vi "ASM.StateExecution.vi"(8 "error in (no error)":errorcluster, 11 "ActorStateMachine in":refnum<class "ActorStateMachine.lvclass">) -> (0 "error out":errorcluster, 3 "ActorStateMachine out":refnum<class "ActorStateMachine.lvclass">)   [LabVIEW 2021, in "ActorStateMachine.lvlib" / "ActorStateMachine.lvclass"]
uses:
  ActorStateMachine.lvclass
  ActorStateMachine.lvclass/ActorStateMachine.ctl
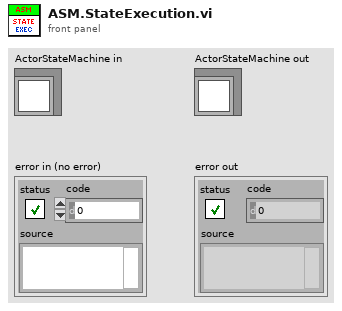
[diagram p1: front panel]
types:
  T1 = typedef "ActorStateMachine.lvlib/ActorStateMachine.lvclass/_ASM.State.ctl" = enum16{"Boom", "Pre-Init", "Init", "Post-Init", "Pre-Reset", "Reset", "Post-Reset", "Pre-Config", "Config", "Post-Config", "Pre-Ready", "Ready", "Post-Ready", "Pre-Running", "Running", "Next", "Post-Running", "Break", "Fail", "Crash", "Shutdown", "Doom"}
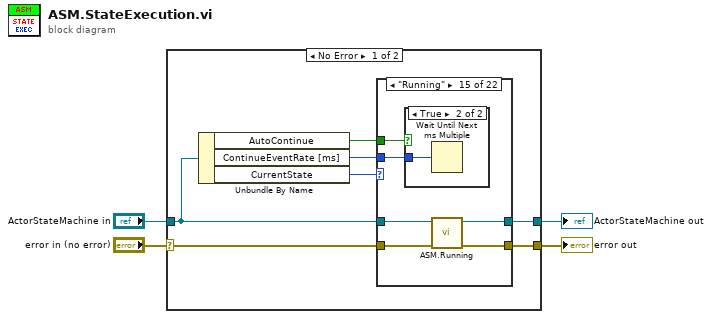
[diagram p0: block diagram]
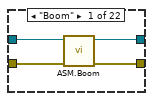
[diagram p2: hidden frame]
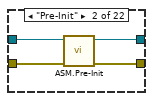
[diagram p3: hidden frame]
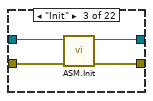
[diagram p4: hidden frame]
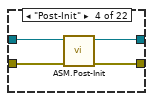
[diagram p5: hidden frame]
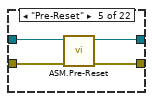
[diagram p6: hidden frame]
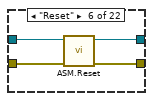
[diagram p7: hidden frame]
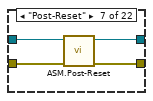
[diagram p8: hidden frame]
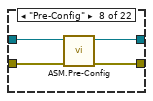
[diagram p9: hidden frame]
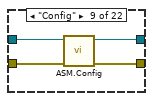
[diagram p10: hidden frame]
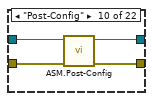
[diagram p11: hidden frame]
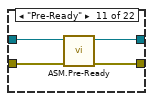
[diagram p12: hidden frame]
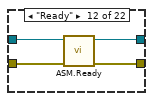
[diagram p13: hidden frame]
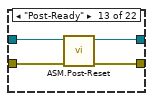
[diagram p14: hidden frame]
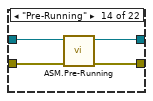
[diagram p15: hidden frame]
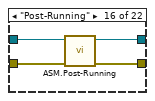
[diagram p17: hidden frame]
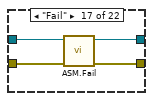
[diagram p18: hidden frame]
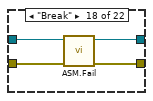
[diagram p19: hidden frame]
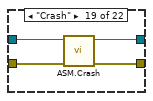
[diagram p20: hidden frame]
diagram:
  n1 = case shown="No Error" "error in (no error)" {
    selector: "error in (no error)" -> [w8 w102]
    tunnel: [w7 w102] -> w3
    tunnel: [w10 w101] -> w1
    tunnel: "ActorStateMachine in" -> [w9 w101]
    frame No Error {
      n2 = Unbundle By Name(w9) -> ("AutoContinue"=w5:bool, "ContinueEventRate [ms]"=w6:u32, "CurrentState"=w11:T1)
      n3 = case shown="\"Running\"" w11 {
        tunnel: [w14 w18 w23 w26 w30 w34 w38 w42 w46 w50 w54 w58 w62 w66 w70 w77 w81 w85 w89 w93 w97 w99] -> w7
        tunnel: [w12 w16 w21 w24 w28 w32 w36 w40 w44 w48 w52 w56 w60 w64 w71 w75 w79 w83 w87 w91 w95 w100] -> w10
        tunnel: w9 -> [w13 w17 w22 w25 w29 w33 w37 w41 w45 w49 w53 w57 w61 w65 w72 w76 w80 w84 w88 w92 w96 w100]
        tunnel: w8 -> [w15 w19 w20 w27 w31 w35 w39 w43 w47 w51 w55 w59 w63 w67 w73 w78 w82 w86 w90 w94 w98 w99]
        tunnel: w6 -> [_ _ _ _ _ _ _ _ _ _ _ _ _ _ w69 _ _ _ _ _ _ _]
        tunnel: w5 -> [_ _ _ _ _ _ _ _ _ _ _ _ _ _ w68 _ _ _ _ _ _ _]
        frame "Boom" {
          n4 = call-dynamic "ASM.Boom.vi"("error in (no error)"=w15, "ActorStateMachine in"=w13) -> ("error out"=w14:errorcluster, "ActorStateMachine out"=w12:refnum<class "ActorStateMachine.lvclass">)  [unwired: 8 in]
        }
        frame "Pre-Init" {
          n5 = call-dynamic "ASM.Pre-Init.vi"("error in (no error)"=w19, "ActorStateMachine in"=w17) -> ("error out"=w18:errorcluster, "ActorStateMachine out"=w16:refnum<class "ActorStateMachine.lvclass">)  [unwired: 8 in]
        }
        frame "Init" {
          n6 = call-dynamic "ASM.Init.vi"("error in (no error)"=w20, "ActorStateMachine in"=w22) -> ("error out"=w23:errorcluster, "ActorStateMachine out"=w21:refnum<class "ActorStateMachine.lvclass">)  [unwired: 8 in]
        }
        frame "Post-Init" {
          n7 = call-dynamic "ASM.Post-Init.vi"("error in (no error)"=w27, "ActorStateMachine in"=w25) -> ("error out"=w26:errorcluster, "ActorStateMachine out"=w24:refnum<class "ActorStateMachine.lvclass">)  [unwired: 8 in]
        }
        frame "Pre-Reset" {
          n8 = call-dynamic "ASM.Pre-Reset.vi"("error in (no error)"=w31, "ActorStateMachine in"=w29) -> ("error out"=w30:errorcluster, "ActorStateMachine out"=w28:refnum<class "ActorStateMachine.lvclass">)  [unwired: 8 in]
        }
        frame "Reset" {
          n9 = call-dynamic "ASM.Reset.vi"("error in (no error)"=w35, "ActorStateMachine in"=w33) -> ("error out"=w34:errorcluster, "ActorStateMachine out"=w32:refnum<class "ActorStateMachine.lvclass">)  [unwired: 8 in]
        }
        frame "Post-Reset" {
          n10 = call-dynamic "ASM.Post-Reset.vi"("error in (no error)"=w39, "ActorStateMachine in"=w37) -> ("error out"=w38:errorcluster, "ActorStateMachine out"=w36:refnum<class "ActorStateMachine.lvclass">)  [unwired: 8 in]
        }
        frame "Pre-Config" {
          n11 = call-dynamic "ASM.Pre-Config.vi"("error in (no error)"=w43, "ActorStateMachine in"=w41) -> ("error out"=w42:errorcluster, "ActorStateMachine out"=w40:refnum<class "ActorStateMachine.lvclass">)  [unwired: 8 in]
        }
        frame "Config" {
          n12 = call-dynamic "ASM.Config.vi"("error in (no error)"=w47, "ActorStateMachine in"=w45) -> ("error out"=w46:errorcluster, "ActorStateMachine out"=w44:refnum<class "ActorStateMachine.lvclass">)  [unwired: 8 in]
        }
        frame "Post-Config" {
          n13 = call-dynamic "ASM.Post-Config.vi"("error in (no error)"=w51, "ActorStateMachine in"=w49) -> ("error out"=w50:errorcluster, "ActorStateMachine out"=w48:refnum<class "ActorStateMachine.lvclass">)  [unwired: 8 in]
        }
        frame "Pre-Ready" {
          n14 = call-dynamic "ASM.Pre-Ready.vi"("error in (no error)"=w55, "ActorStateMachine in"=w53) -> ("error out"=w54:errorcluster, "ActorStateMachine out"=w52:refnum<class "ActorStateMachine.lvclass">)  [unwired: 8 in]
        }
        frame "Ready" {
          n15 = call-dynamic "ASM.Ready.vi"("error in (no error)"=w59, "ActorStateMachine in"=w57) -> ("error out"=w58:errorcluster, "ActorStateMachine out"=w56:refnum<class "ActorStateMachine.lvclass">)  [unwired: 8 in]
        }
        frame "Post-Ready" {
          n16 = call-dynamic "ASM.Post-Reset.vi"("error in (no error)"=w63, "ActorStateMachine in"=w61) -> ("error out"=w62:errorcluster, "ActorStateMachine out"=w60:refnum<class "ActorStateMachine.lvclass">)  [unwired: 8 in]
        }
        frame "Pre-Running" {
          n17 = call-dynamic "ASM.Pre-Running.vi"("error in (no error)"=w67, "ActorStateMachine in"=w65) -> ("error out"=w66:errorcluster, "ActorStateMachine out"=w64:refnum<class "ActorStateMachine.lvclass">)  [unwired: 8 in]
        }
        frame "Running" {
          n18 = case shown="True" w68 {
            tunnel: w69 -> [_ w74]
            frame False {
            }
            frame True {
              n19 = Wait Until Next ms Multiple(millisecond multiple=w74) -> ()  [unwired: 1 out]
            }
          }
          n20 = call-dynamic "ASM.Running.vi"("error in (no error)"=w73, "ActorStateMachine in"=w72) -> ("error out"=w70:errorcluster, "ActorStateMachine out"=w71:refnum<class "ActorStateMachine.lvclass">)  [unwired: 8 in]
        }
        frame "Post-Running" {
          n21 = call-dynamic "ASM.Post-Running.vi"("error in (no error)"=w78, "ActorStateMachine in"=w76) -> ("error out"=w77:errorcluster, "ActorStateMachine out"=w75:refnum<class "ActorStateMachine.lvclass">)  [unwired: 8 in]
        }
        frame "Fail" {
          n22 = call-dynamic "ASM.Fail.vi"("error in (no error)"=w82, "ActorStateMachine in"=w80) -> ("error out"=w81:errorcluster, "ActorStateMachine out"=w79:refnum<class "ActorStateMachine.lvclass">)  [unwired: 8 in]
        }
        frame "Break" {
          n23 = call-dynamic "ASM.Fail.vi"("error in (no error)"=w86, "ActorStateMachine in"=w84) -> ("error out"=w85:errorcluster, "ActorStateMachine out"=w83:refnum<class "ActorStateMachine.lvclass">)  [unwired: 8 in]
        }
        frame "Crash" {
          n24 = call-dynamic "ASM.Crash.vi"("error in (no error)"=w90, "ActorStateMachine in"=w88) -> ("error out"=w89:errorcluster, "ActorStateMachine out"=w87:refnum<class "ActorStateMachine.lvclass">)  [unwired: 8 in]
        }
        frame "Shutdown" {
          n25 = call-dynamic "ASM.Shutdown.vi"("error in (no error)"=w94, "ActorStateMachine in"=w92) -> ("error out"=w93:errorcluster, "ActorStateMachine out"=w91:refnum<class "ActorStateMachine.lvclass">)  [unwired: 8 in]
        }
        frame "Doom" {
          n26 = call-dynamic "ASM.Doom.vi"("error in (no error)"=w98, "ActorStateMachine in"=w96) -> ("error out"=w97:errorcluster, "ActorStateMachine out"=w95:refnum<class "ActorStateMachine.lvclass">)  [unwired: 8 in]
        }
        frame Default {
        }
      }
    }
    frame Error {
    }
  }
  "error out" <- w3
  "ActorStateMachine out" <- w1
